vi "PR_Update_screw_information .vi"(7 "鎖螺絲DATA":T1, 8 "error in (no error)":errorcluster, 10 "barcode":string="123465798", 11 "DBlink":string="Driver={ODBC Driver 17 for SQL Server};Server=localhost\\SQLEXPRESS;Database=ZDX201;UID=labview;PWD=Dsa@54137926") -> (0 "error out":errorcluster, 2 "screw_result":string)   [LabVIEW 2019]
uses:
  <vilib>/addons/database/Auxilliary.llb/DB Tools Format Datetime String (Time Stamp).vi
  <vilib>/addons/database/Connection.llb/DB Tools Open Connec (String).vi
  <vilib>/addons/database/NI_Database_API.lvlib
panel:
  out "concatenated string":string="WHERE [barcode]='123465798' and [position]='A'"
  # "視覺判定結果\n0. 未拍攝(S08）\n1. OK無異常\n2. PIN無對正(S09)\n3. PCB未放正(S10)\n4(預設). 其他(S07)"
  # "各個螺絲的判定結果\n0. 未鎖附(S01~S06）\n1. OK (有鎖但是扭力沒到達S11~S16)\n2. NG (有鎖但是NG，S21~S26）\n3. 空轉(第三次排出，S31~S36）\n4. 滑牙(排出，S41~S46）\n5(預設). 其他"
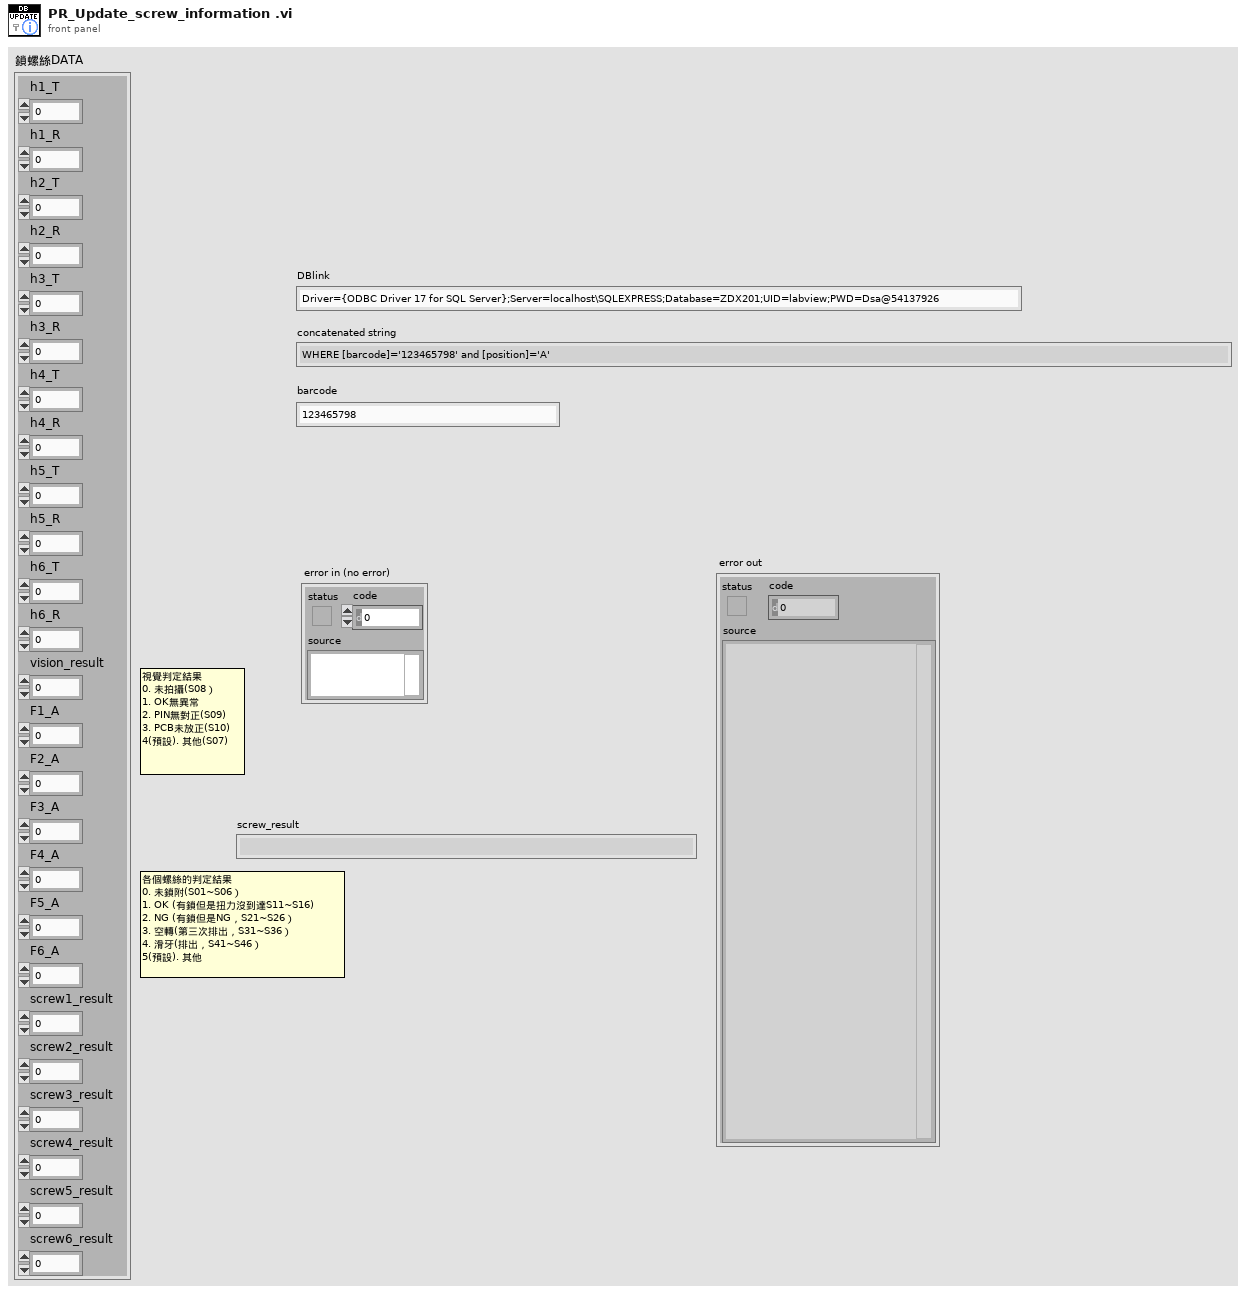
[diagram p1: front panel]
types:
  T1 = cluster{"h1_T":dbl, "h1_R":dbl, "h2_T":dbl, "h2_R":dbl, "h3_T":dbl, "h3_R":dbl, "h4_T":dbl, "h4_R":dbl, "h5_T":dbl, "h5_R":dbl, "h6_T":dbl, "h6_R":dbl, "vision_result":i32, "F1_A":dbl, "F2_A":dbl, "F3_A":dbl, "F4_A":dbl, "F5_A":dbl, "F6_A":dbl, "screw1_result":i32, "screw2_result":i32, "screw3_result":i32, "screw4_result":i32, "screw5_result":i32, "screw6_result":i32}
  T2 = cluster{"h1_T":dbl, "h1_R":dbl, "h2_T":dbl, "h2_R":dbl, "h3_T":dbl, "h3_R":dbl, "h4_T":dbl, "h4_R":dbl, "h5_T":dbl, "h5_R":dbl, "h6_T":dbl, "h6_R":dbl, "screw_result":string, "update_time":timestamp, "F1_A":dbl, "F2_A":dbl, "F3_A":dbl, "F4_A":dbl, "F5_A":dbl, "F6_A":dbl}
  T3 = typedef "NI_Database_API.lvlib/Conn ObjectReference.ctl" = refnum<k1>
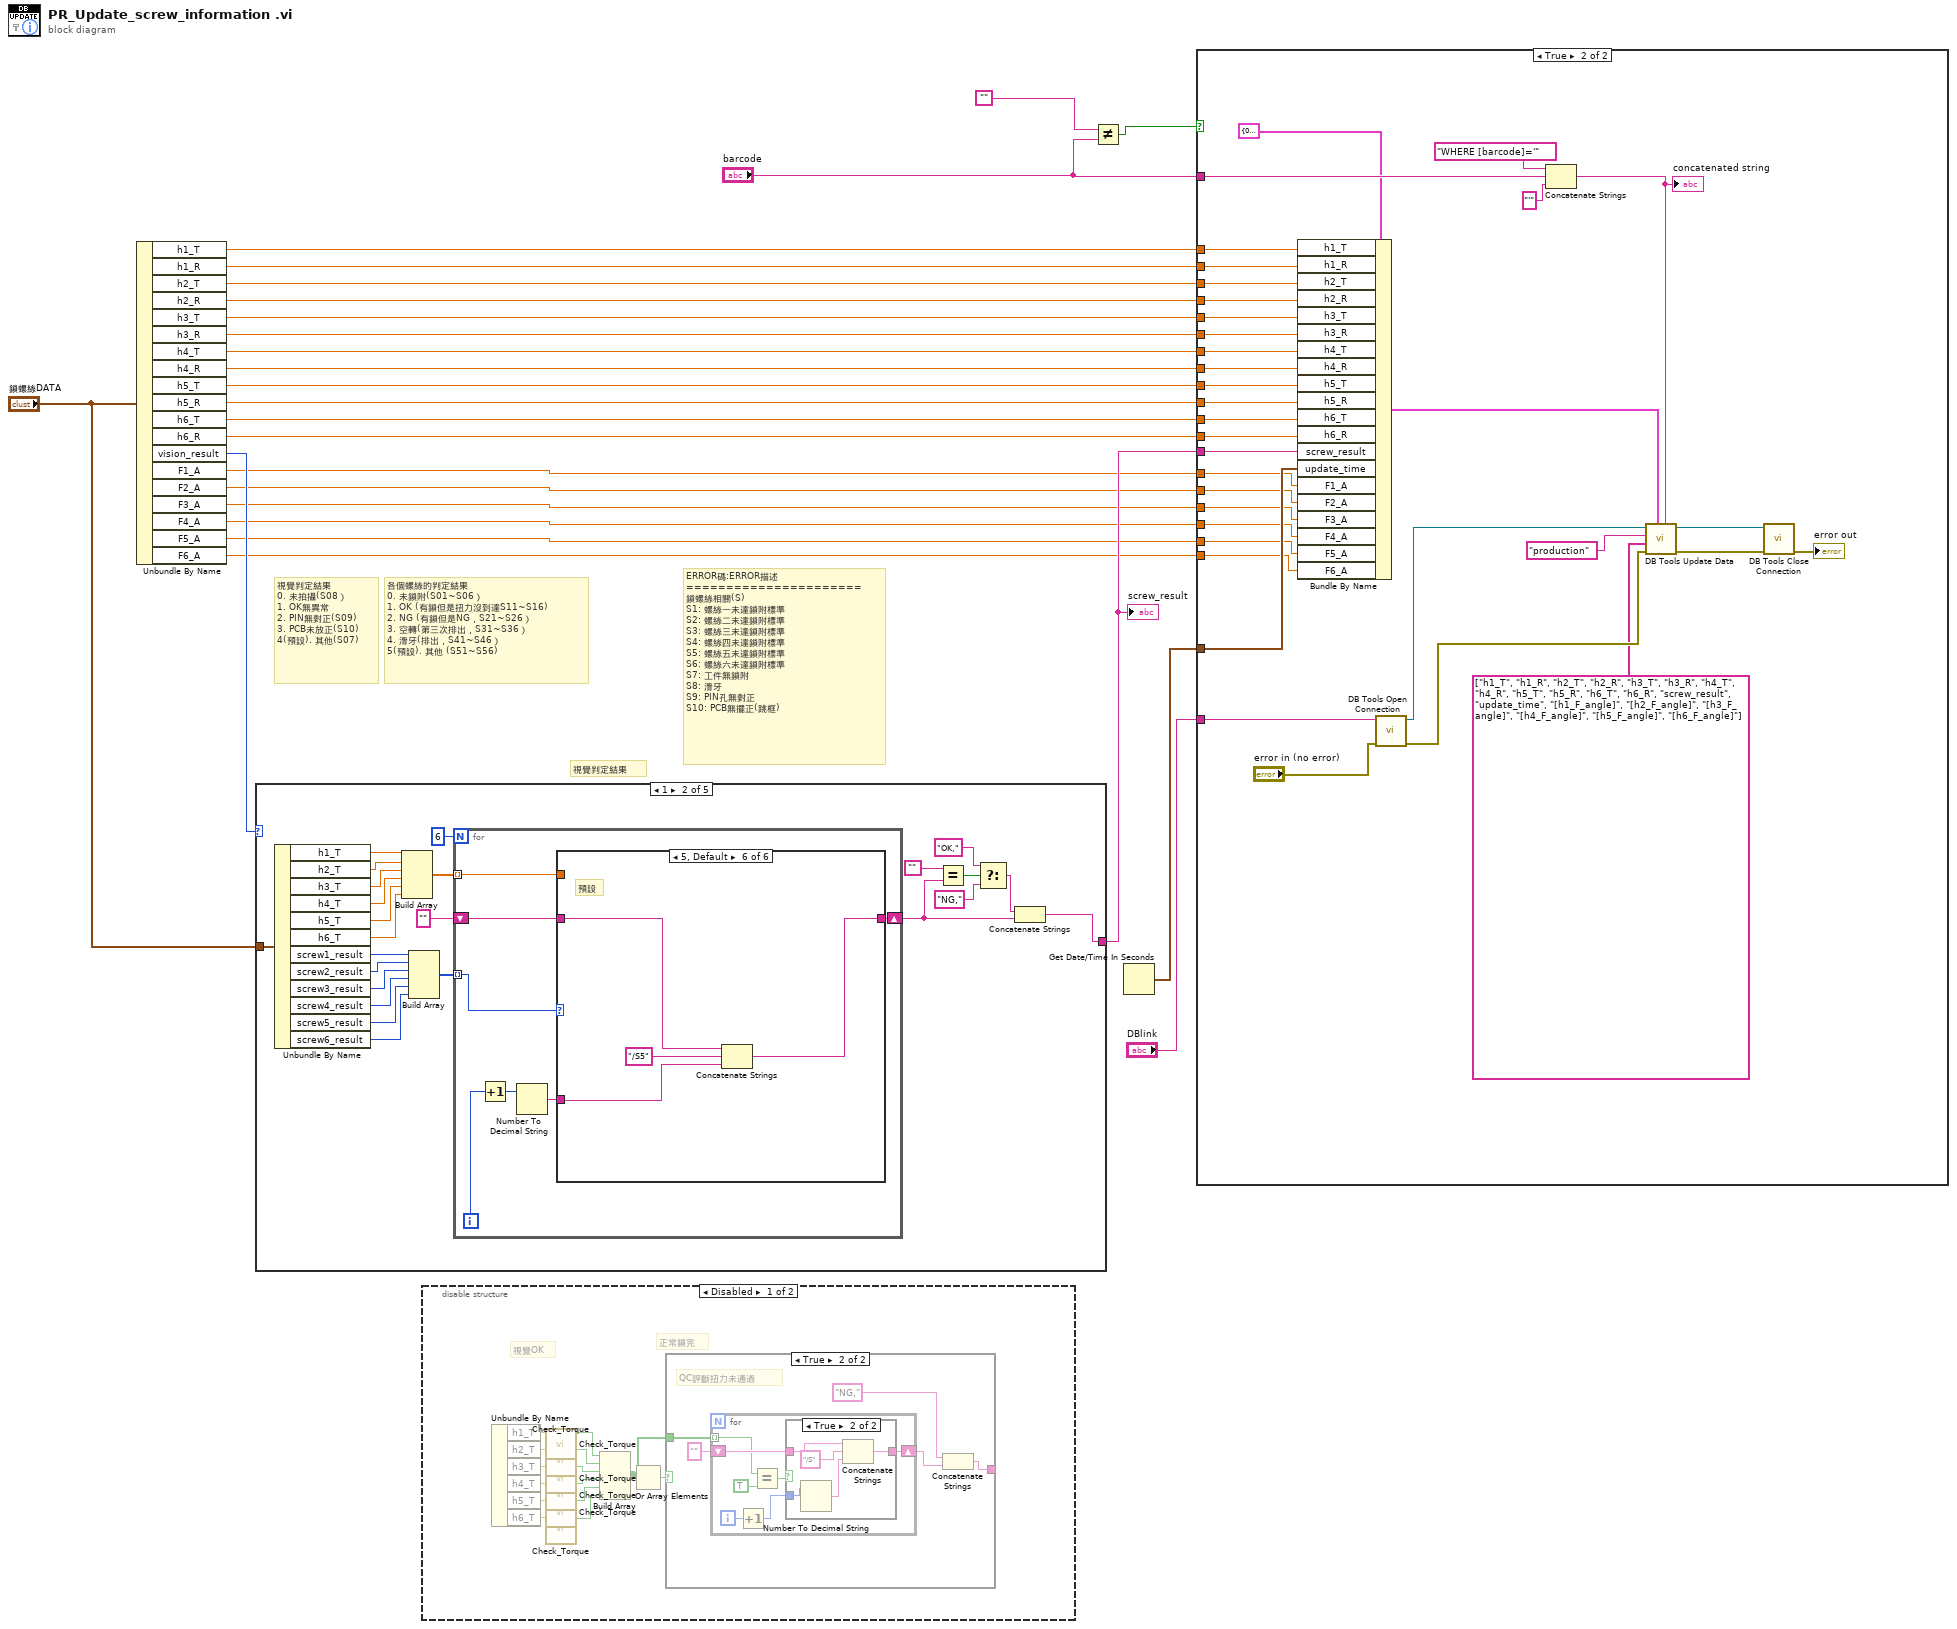
[diagram p0: block diagram]
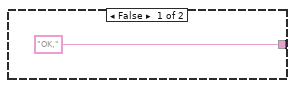
[diagram p2: hidden frame]
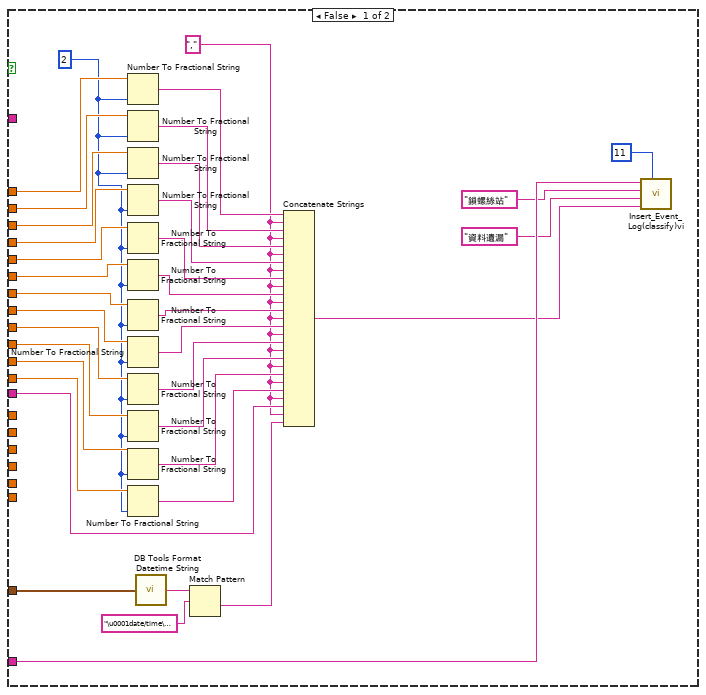
[diagram p5: hidden frame]
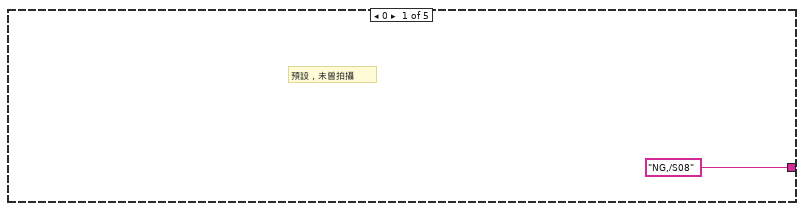
[diagram p6: hidden frame]
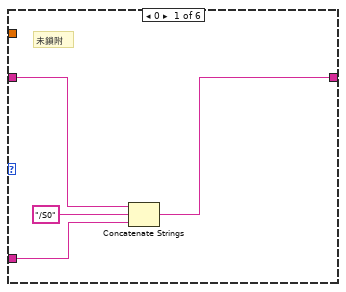
[diagram p7: hidden frame]
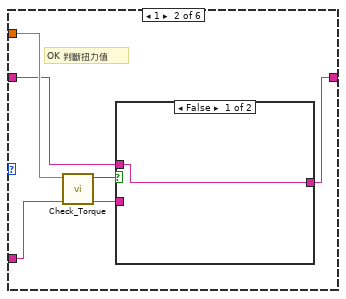
[diagram p8: hidden frame]
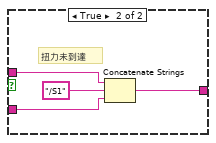
[diagram p9: hidden frame]
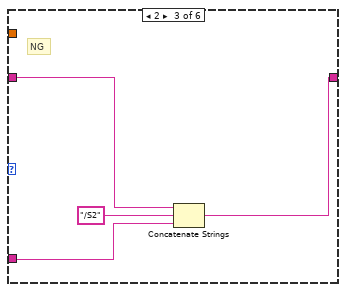
[diagram p10: hidden frame]
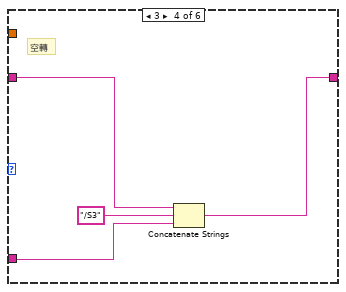
[diagram p11: hidden frame]
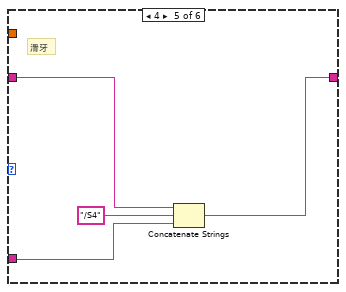
[diagram p12: hidden frame]
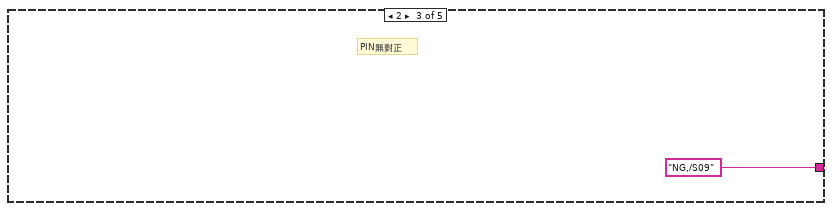
[diagram p13: hidden frame]
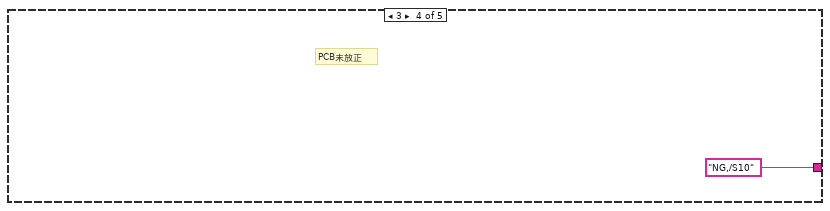
[diagram p14: hidden frame]
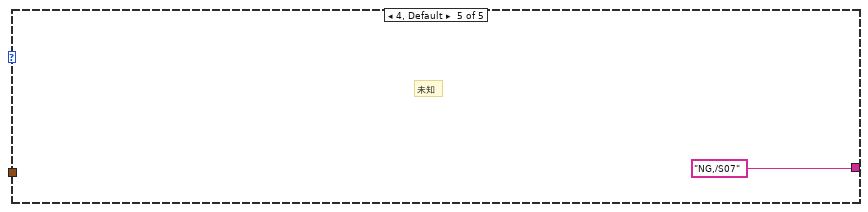
[diagram p15: hidden frame]
diagram:
  # "視覺判定結果"
  # "視覺判定結果\n0. 未拍攝(S08）\n1. OK無異常\n2. PIN無對正(S09)\n3. PCB未放正(S10)\n4(預設). 其他(S07)"
  # "各個螺絲的判定結果\n0. 未鎖附(S01~S06）\n1. OK (有鎖但是扭力沒到達S11~S16)\n2. NG (有鎖但是NG，S21~S26）\n3. 空轉(第三次排出，S31~S36）\n4. 滑牙(排出，S41~S46）\n5(預設). 其他 (S51~S56)"
  # "ERROR碼:ERROR描述\n======================\n鎖螺絲相關(S)\nS1: 螺絲一未達鎖附標準\nS2: 螺絲二未達鎖附標準\nS3: 螺絲三未達鎖附標準\nS4: 螺絲四未達鎖附標準\nS5: 螺絲五未達鎖附標準\nS6: 螺絲六未達鎖附標準\nS7: 工件無鎖附\nS8: 滑牙\nS9: PIN孔無對正\nS10: PCB無擺正(跳框)"
  n1 = Unbundle By Name("鎖螺絲DATA") -> ("h1_T"=w25:dbl, "h1_R"=w24:dbl, "h2_T"=w23:dbl, "h2_R"=w22:dbl, "h3_T"=w21:dbl, "h3_R"=w20:dbl, "h4_T"=w19:dbl, "h4_R"=w18:dbl, "h5_T"=w17:dbl, "h5_R"=w16:dbl, "h6_T"=w15:dbl, "h6_R"=w14:dbl, "vision_result"=w12:i32, "F1_A"=w7:dbl, "F2_A"=w6:dbl, "F3_A"=w5:dbl, "F4_A"=w4:dbl, "F5_A"=w3:dbl, "F6_A"=w2:dbl)
  n2 = case shown="1" w12 {
    tunnel: ["NG,/S08" ("screw_result") w28 "NG,/S09" ("screw_result") "NG,/S10" ("screw_result") "NG,/S07" ("screw_result")] -> w11
    tunnel: "鎖螺絲DATA" -> [_ w50 _ _ _]
    frame 0 {
      # "預設，未曾拍攝"
    }
    frame 1 {
      n3 = Unbundle By Name(w50) -> ("h1_T"=w49:dbl, "h2_T"=w48:dbl, "h3_T"=w47:dbl, "h4_T"=w46:dbl, "h5_T"=w45:dbl, "h6_T"=w44:dbl, "screw1_result"=w43:i32, "screw2_result"=w42:i32, "screw3_result"=w41:i32, "screw4_result"=w40:i32, "screw5_result"=w39:i32, "screw6_result"=w38:i32)
      n4 = Build Array(w49, w48, w47, w46, w45, w44) -> (w36:dbl[])
      n5 = Build Array(w43, w42, w41, w40, w39, w38) -> (w37:i32[])
      n6 = for {
        N: 6 -> [_]
        tunnel: w37 -> [w58] mode=indexing
        tunnel: w36 -> [w52] mode=indexing
        shift-right: [w53] -> w29
        shift-left: "" -> [w54]
        i -> [w56]
        n7 = Increment(x=w56) -> (x+1=w57:i32)
        n8 = Number To Decimal String(number=w57) -> (decimal integer string=w55:string)  [unwired: 1 in]
        n9 = case shown="5, Default" w58 {
          tunnel: w55 -> [w61 w65 w75 w79 w83 w87]
          tunnel: w54 -> [w60 w64 w74 w78 w82 w86]
          tunnel: [w59 w63 w73 w77 w81 w85] -> w53
          tunnel: w52 -> [_ w67 _ _ _ _]
          frame 0 {
            # "未鎖附"
            n10 = Concatenate Strings(w60, "/S0", w61) -> (w59:string)
          }
          frame 1 {
            # "OK 判斷扭力值"
            n11 = call "Check_Torque.vi"("Torque"=w67) -> ("Pass/ Failure?"=w66:bool)  [unwired: 10 in]
            n12 = case shown="False" w66 {
              tunnel: w65 -> [_ w71]
              tunnel: w64 -> [w68 w70]
              tunnel: [w68 w69] -> w63
              frame False {
              }
              frame True {
                # "扭力未到達"
                n13 = Concatenate Strings(w70, "/S1", w71) -> (w69:string)
              }
            }
          }
          frame 2 {
            # "NG"
            n14 = Concatenate Strings(w74, "/S2", w75) -> (w73:string)
          }
          frame 3 {
            # "空轉"
            n15 = Concatenate Strings(w78, "/S3", w79) -> (w77:string)
          }
          frame 4 {
            # "滑牙"
            n16 = Concatenate Strings(w82, "/S4", w83) -> (w81:string)
          }
          frame 5, Default {
            # "預設"
            n17 = Concatenate Strings(w86, "/S5", w87) -> (w85:string)
          }
        }
      }
      n18 = Equal?(x="", y=w29) -> (x = y?=w34:bool)
      n19 = Select(t="OK," ("screw_result"), s=w34, f="NG," ("screw_result")) -> (s? t:f=w30:string)
      n20 = Concatenate Strings(w30, w29) -> (w28:string)
    }
    frame 2 {
      # "PIN無對正"
    }
    frame 3 {
      # "PCB未放正"
    }
    frame 4, Default {
      # "未知"
    }
  }
  "screw_result" <- w11
  n21 = disable-structure shown="Disabled" {
    frame Disabled {
      # "視覺OK"
      # "正常鎖完"
      n22 = Unbundle By Name() -> ("h1_T"=w97:dbl, "h2_T"=w96:dbl, "h3_T"=w95:dbl, "h4_T"=w94:dbl, "h5_T"=w93:dbl, "h6_T"=w92:dbl)  [unwired: 1 in]
      n23 = call "Check_Torque.vi"("Torque"=w97) -> ("Pass/ Failure?"=w98:bool)  [unwired: 10 in]
      n24 = call "Check_Torque.vi"("Torque"=w96) -> ("Pass/ Failure?"=w99:bool)  [unwired: 10 in]
      n25 = call "Check_Torque.vi"("Torque"=w95) -> ("Pass/ Failure?"=w100:bool)  [unwired: 10 in]
      n26 = call "Check_Torque.vi"("Torque"=w94) -> ("Pass/ Failure?"=w101:bool)  [unwired: 10 in]
      n27 = call "Check_Torque.vi"("Torque"=w93) -> ("Pass/ Failure?"=w102:bool)  [unwired: 10 in]
      n28 = call "Check_Torque.vi"("Torque"=w92) -> ("Pass/ Failure?"=w103:bool)  [unwired: 10 in]
      n29 = Build Array(w98, w99, w100, w101, w102, w103) -> (w105:bool[])
      n30 = Or Array Elements(Boolean array=w105) -> (logical OR=w104:bool)
      n31 = case shown="True" w104 {
        tunnel: ["OK," ("screw_result") w109] -> _
        tunnel: w105 -> [_ w111]
        frame False {
        }
        frame True {
          # "QC評斷扭力未通過"
          n32 = for {
            tunnel: w111 -> [w116] mode=indexing
            shift-right: [w112] -> w110
            shift-left: "" -> [w118]
            i -> [w114]
            n33 = Increment(x=w114) -> (x+1=w113:i32)
            n34 = Equal?(x=w116, y=TRUE) -> (x = y?=w115:bool)
            n35 = case shown="True" w115 {
              tunnel: w118 -> [w119 w124]
              tunnel: w113 -> [_ w122]
              tunnel: [w119 w120] -> w112
              frame False {
              }
              frame True {
                n36 = Number To Decimal String(number=w122) -> (decimal integer string=w121:string)  [unwired: 1 in]
                n37 = Concatenate Strings(w124, "/S" ("string"), w121) -> (w120:string)
              }
            }
          }
          n38 = Concatenate Strings("NG,", w110) -> (w109:string)
        }
      }
    }
    frame Enabled {
    }
  }
  n39 = Not Equal?(x="", y="barcode") -> (x != y?=w10:bool)
  n40 = Get Date/Time In Seconds() -> (seconds since 1Jan1904=w13:timestamp)
  n41 = case shown="True" w10 {
    tunnel: "DBlink" -> [w160 w189]
    tunnel: "barcode" -> [_ w185]
    tunnel: w25 -> [w156 w182]
    tunnel: w24 -> [w155 w181]
    tunnel: w23 -> [w154 w180]
    tunnel: w22 -> [w153 w179]
    tunnel: w21 -> [w152 w178]
    tunnel: w20 -> [w151 w177]
    tunnel: w19 -> [w150 w176]
    tunnel: w18 -> [w149 w175]
    tunnel: w17 -> [w148 w174]
    tunnel: w16 -> [w147 w173]
    tunnel: w15 -> [w146 w172]
    tunnel: w14 -> [w145 w171]
    tunnel: w13 -> [w128 w169]
    tunnel: w11 -> [w132 w168]
    tunnel: w7 -> [_ w166]
    tunnel: w6 -> [_ w165]
    tunnel: w5 -> [_ w164]
    tunnel: w4 -> [_ w163]
    tunnel: w3 -> [_ w162]
    tunnel: w2 -> [_ w161]
    frame False {
      w125 = i16 2 ("precision (6)")
      w131 = "," ("string")
      n42 = Number To Fractional String(number=w156, precision (6)=w125) -> (F-format string=w144:string)  [unwired: 2 in]
      n43 = Number To Fractional String(number=w155, precision (6)=w125) -> (F-format string=w143:string)  [unwired: 2 in]
      n44 = Number To Fractional String(number=w154, precision (6)=w125) -> (F-format string=w142:string)  [unwired: 2 in]
      n45 = Number To Fractional String(number=w153, precision (6)=w125) -> (F-format string=w141:string)  [unwired: 2 in]
      n46 = Number To Fractional String(number=w152, precision (6)=w125) -> (F-format string=w140:string)  [unwired: 2 in]
      n47 = Number To Fractional String(number=w151, precision (6)=w125) -> (F-format string=w139:string)  [unwired: 2 in]
      n48 = Number To Fractional String(number=w150, precision (6)=w125) -> (F-format string=w138:string)  [unwired: 2 in]
      n49 = Number To Fractional String(number=w149, precision (6)=w125) -> (F-format string=w137:string)  [unwired: 2 in]
      n50 = Number To Fractional String(number=w148, precision (6)=w125) -> (F-format string=w136:string)  [unwired: 2 in]
      n51 = Number To Fractional String(number=w147, precision (6)=w125) -> (F-format string=w135:string)  [unwired: 2 in]
      n52 = Number To Fractional String(number=w146, precision (6)=w125) -> (F-format string=w134:string)  [unwired: 2 in]
      n53 = Number To Fractional String(number=w145, precision (6)=w125) -> (F-format string=w133:string)  [unwired: 2 in]
      n54 = call-poly <vilib>:"DB Tools Format Datetime String.vi"("time stamp"=w128) -> ("date/time string"=w129:string)
      n55 = Match Pattern(string=w129, regular expression="\u0001date/time\u0001" ("search string")) -> (after substring=w127:string)  [unwired: 1 in, 3 out]
      n56 = Concatenate Strings(w144, w131, w143, w131, w142, w131, w141, w131, w140, w131, w139, w131, w138, w131, w137, w131, w136, w131, w135, w131, w134, w131, w133, w131, w132, w131, w127) -> (w126:string)
      n57 = call "Insert_Event_Log(classify)vi.vi"("classify"=i16 11, "data"=w126, "message"="資料遺漏", "id"="鎖螺絲站", "DBlink"=w160) -> ()  [unwired: 6 in, 1 out]
    }
    frame True {
      n58 = Bundle By Name(cluster=T2 {"h1_T"=0.0, "h1_R"=0.0, "h2_T"=0.0, "h2_R"=0.0, "h3_T"=0.0, "h3_R"=0.0, "h4_T"=0.0, "h4_R"=0.0, "h5_T"=0.0, "h5_R"=0.0, "h6_T"=0.0, "h6_R"=0.0, "screw_result"="", "update_time"=timestamp(0 s since 1904-01-01), "F1_A"=0.0, "F2_A"=0.0, "F3_A"=0.0, "F4_A"=0.0, "F5_A"=0.0, "F6_A"=0.0} ("鎖螺絲DATA"), "h1_T"=w182, "h1_R"=w181, "h2_T"=w180, "h2_R"=w179, "h3_T"=w178, "h3_R"=w177, "h4_T"=w176, "h4_R"=w175, "h5_T"=w174, "h5_R"=w173, "h6_T"=w172, "h6_R"=w171, "screw_result"=w168, "update_time"=w169, "F1_A"=w166, "F2_A"=w165, "F3_A"=w164, "F4_A"=w163, "F5_A"=w162, "F6_A"=w161) -> (w170:T2)
      n59 = call-poly <vilib>:"DB Tools Open Connection.vi"("error in (no error)"="error in (no error)", "connection information"=w189) -> ("error out"=w193:errorcluster, "connection reference"=w191:T3)  [unwired: 6 in]
      n60 = Concatenate Strings("WHERE [barcode]='", w185, "'" ("string")) -> (w186:string)
      "concatenated string" <- w186
      n61 = call <vilib>:"DB Tools Update Data.vi"("condition"=w186, "data"=w170, "error in (no error)"=w193, "columns"=string[] ["h1_T", "h1_R", "h2_T", "h2_R", "h3_T", "h3_R", "h4_T", "h4_R", "h5_T", "h5_R", "h6_T", "h6_R", "screw_result", "update_time", "[h1_F_angle]", "[h2_F_angle]", "[h3_F_angle]", "[h4_F_angle]", "[h5_F_angle]", "[h6_F_angle]"] ("columns 2"), "table"="production", "connection reference"=w191) -> ("error out"=w194:errorcluster, "connection reference out"=w192:T3)  [unwired: 4 in]
      n62 = call <vilib>:"DB Tools Close Connection.vi"("error in (no error)"=w194, "connection reference"=w192) -> ("error out"=→"error out":errorcluster)  [unwired: 5 in]
    }
  }
